vi "start.vi"(8 "error in (no error)":errorcluster, 9 "ILCAppConfig":T1={"ILCConfig"={"Input Channels"=enum."Channel 0", "Scan Rate (Hz) "=enum."50", "ADC PGA Gain"=0}, "SerialConfig"={"VISA resource name"="", "Baud Rate"=9600, "Data Bits"=8, "Parity"=enum."None", "Stop Bits"=10, "Flow Control"=0, "Timeout (ms)"=10000, "Serial Protocol"=enum."RS485"}, "Application Timing"={"Loop Period (ms)"=1}} {"Application Timing"."Loop Period (ms)" min=1 max=5000; "SerialConfig"."Stop Bits" items=["1.0"=10, "1.5"=15, "2.0"=20]; "SerialConfig"."Flow Control" items=["None", "XON/XOFF", "RTS/CTS", "XON/XOFF & RTS/CTS", "DTR/DSR", "XON/XOFF & DTR/DSR"]; "SerialConfig"."Data Bits" min=5 max=8 step=1; "ILCConfig"."ADC PGA Gain" max=7}, 10 "model":refnum<class "Model.lvclass">, 11 "State in":refnum<class "State.lvclass">) -> (0 "error out":errorcluster, 2 "model 2":refnum<class "Model.lvclass">, 3 "State out":refnum<class "State.lvclass">)   [LabVIEW 2012, in "State.lvclass"]
uses:
  State.lvclass
  Model/Model/Model.lvclass
  ILCAppConfig.ctl
  Program Files (x86)/National Instruments/LabVIEW 2012/user.lib/Common/ILC/Configuration/ILCConfig.ctl
  Program Files (x86)/National Instruments/LabVIEW 2012/user.lib/Common/ILC/Configuration/InputChannels.ctl
  Program Files (x86)/National Instruments/LabVIEW 2012/user.lib/Common/ILC/Configuration/ScanRate_Hz_MultichannelOptions.ctl
  Program Files (x86)/National Instruments/LabVIEW 2012/user.lib/Common/SerialProtocols/Configuration/SerialConfig.ctl
  Program Files (x86)/National Instruments/LabVIEW 2012/user.lib/Common/SerialProtocols/Configuration/SerialProtocol.ctl
  Program Files (x86)/National Instruments/LabVIEW 2012/user.lib/Common/Component/Application/Configuration/ApplicationTiming.ctl
  Program Files (x86)/National Instruments/LabVIEW 2012/user.lib/Common/ILC/Configuration/ILCConfiguration.lvlib
  Program Files (x86)/National Instruments/LabVIEW 2012/user.lib/Common/SerialProtocols/SerialProtocols.lvlib
  Program Files (x86)/National Instruments/LabVIEW 2012/user.lib/Common/Component/Application/Application.lvlib
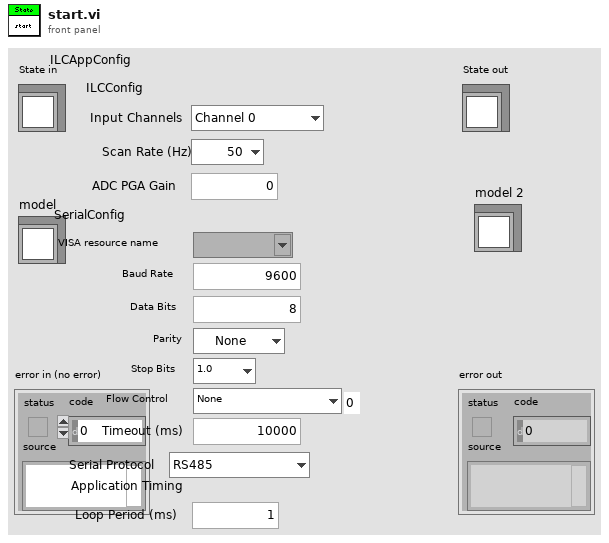
[diagram p1: front panel]
types:
  T1 = typedef "ILCAppConfig.ctl" = cluster{"ILCConfig":T2, "SerialConfig":T5, "Application Timing":T7}
  T2 = typedef "ILCCommon.lvlib/ILCConfiguration.lvlib/ILCConfig.ctl" = cluster{"Input Channels":T3, "Scan Rate (Hz) ":T4, "ADC PGA Gain":u8}
  T3 = typedef "ILCCommon.lvlib/ILCConfiguration.lvlib/InputChannels.ctl" = enum16{"Channel 0", "3 Channels", "5 Channels"}
  T4 = typedef "ILCCommon.lvlib/ILCConfiguration.lvlib/ScanRate_Hz_MultichannelOptions.ctl" = enum16{"50", "60", "100", "120", "200", "240", "300", "400", "480", "600", "1200", "2400", "4800"}
  T5 = typedef "SerialProtocols.lvlib/SerialConfig.ctl" = cluster{"VISA resource name":refnum<visa-resource-name>, "Baud Rate":u32, "Data Bits":u16, "Parity":enum16{"None", "Odd", "Even", "Mark", "Space"}, "Stop Bits":u16, "Flow Control":u16, "Timeout (ms)":u32, "Serial Protocol":T6}
  T6 = typedef "SerialProtocols.lvlib/SerialProtocol.ctl" = enum16{"RS232", "RS485", "SerialSimulator"}
  T7 = typedef "Application.lvlib/ApplicationTiming.ctl" = cluster{"Loop Period (ms)":u16}
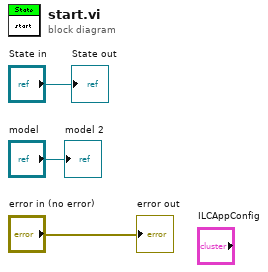
[diagram p0: block diagram]
diagram:
  "error out" <- "error in (no error)"
  "State out" <- "State in"
  "model 2" <- "model"
